vi "Contruct from Settings File.vi"(8 "Error in":errorcluster caption="Error in (no error)", 11 "Settings Path":path) -> (0 "Error out":errorcluster, 3 "Confluence out":refnum<class "Confluence.lvclass">)   [LabVIEW 2023, in "VIDoc Printer - Confluence.lvlib" / "VIDoc Printer - Confluence.lvclass"]
uses:
  VIDoc Printer - Confluence.lvclass
  <userlib>/_PetranWay/LabVIEW Confluence API/Source/Confluence/Confluence Connection/Confluence.lvclass
  <userlib>/_PetranWay/LabVIEW Confluence API/Source/Data Center/Confluence Data Center/Confluence Data Center.lvclass
  C:/Program Files/National Instruments/LabVIEW 2023/user.lib/_PetranWay/LabVIEW Confluence API/Source/Confluence/Confluence Connection/Confluence.lvclass
  <userlib>/_PetranWay/LabVIEW Confluence API/Source/Cloud/Confluence Cloud/Confluence Cloud.lvclass
  <userlib>/_PetranWay/LabVIEW Confluence API/Source/Data Center/Confluence Data Center/API/Construct Confluence Data Center From Cache.vi
  <userlib>/_PetranWay/LabVIEW Confluence API/Source/Cloud/Confluence Cloud/API/Construct Confluence Cloud From Cache.vi
  VIDoc Printer - Confluence.lvclass/VIDoc Printer - Confluence.ctl
  Settings/Confluence Printer Settings/VIDoc Settings - Confluence.lvclass
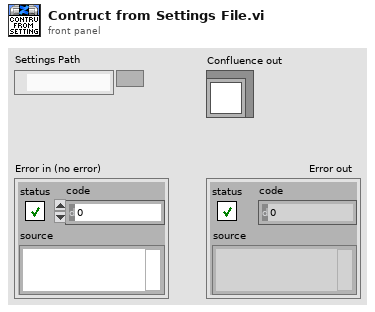
[diagram p1: front panel]
types:
  T1 = typedef "VIDoc Printer - Confluence.lvlib/VIDoc Settings - Confluence.lvclass/Confluence Connection Settings.ctl" = cluster{"Connection Type":enum16{"Data Center", "Cloud"}, "URL":string, "Email":string}
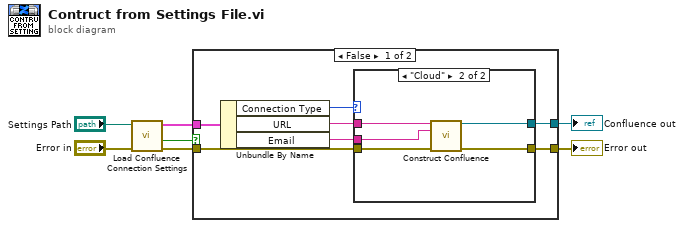
[diagram p0: block diagram]
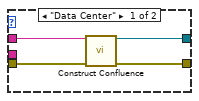
[diagram p2: hidden frame]
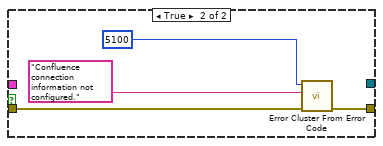
[diagram p3: hidden frame]
diagram:
  n1 = call "Load Confluence Connection Settings.vi"("Error in"="Error in", "Settings Path"="Settings Path") -> ("Error out"=w5:errorcluster, "Loaded Default?"=w4:bool, "Confluence Connection Settings"=w3:T1)  [unwired: 7 in]
  n2 = case shown="False" w4 {
    tunnel: [w14 w26] -> w2
    tunnel: [w13 _] -> w1
    tunnel: w5 -> [w12 w27]
    tunnel: w3 -> [w11 _]
    frame False {
      n3 = Unbundle By Name(w11) -> ("Connection Type"=w10:enum16{"Data Center", "Cloud"}, "URL"=w9:string, "Email"=w8:string)
      n4 = case shown="\"Cloud\"" w10 {
        tunnel: [w18 w23] -> w14
        tunnel: [w17 w22] -> w13
        tunnel: w12 -> [w16 w21]
        tunnel: w9 -> [w15 w20]
        tunnel: w8 -> [_ w19]
        frame "Data Center" {
          n5 = call-poly <userlib>:"Construct Confluence.vi"("Server URL"=w15, "error in (no error)"=w16) -> ("Confluence Data Center out"=w17:refnum<class "Confluence Data Center.lvclass">, "error out"=w18:errorcluster)  [unwired: 10 in, 2 out]
        }
        frame "Cloud" {
          n6 = call-poly <userlib>:"Construct Confluence.vi"("Organization Name (https://[Organization Name].atlassian.net]"=w20, "Email Address"=w19, "error in (no error)"=w21) -> ("Confluence Cloud out"=w22:refnum<class "Confluence Cloud.lvclass">, "error out"=w23:errorcluster)  [unwired: 9 in, 2 out]
        }
      }
    }
    frame True {
      n7 = call <vilib>:"Error Cluster From Error Code.vi"("error in (no error)"=w27, "error message (\"\")"="Confluence connection information not configured." ("error message (\"\")"), "error code (0)"=5100) -> ("error out"=w26:errorcluster)  [unwired: 6 in]
    }
  }
  "Error out" <- w2
  "Confluence out" <- w1
